vi "util-ui-view.vi"(10 "Page2":enum32{"Map", "Editor", "Calibration"}(ring), 11 "Page1":enum32{"MAIN", "I/O", "ADMIN"}(ring)) -> (2 "Pge2 out":string, 3 "Page1 out":string, 5 "Page1:Page2":string)   [LabVIEW 2024]
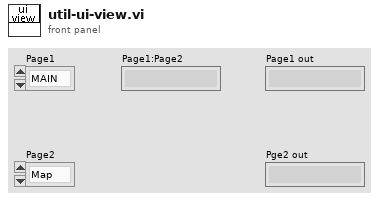
[diagram p1: front panel]
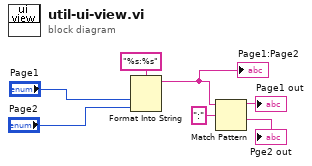
[diagram p0: block diagram]
diagram:
  n1 = Format Into String(format string="%s:%s", "Page1", "Page2") -> (resulting string=w4:string)  [unwired: 2 in, 1 out]
  "Page1:Page2" <- w4
  n2 = Match Pattern(string=w4, regular expression=":") -> (before substring=→"Page1 out":string, after substring=→"Pge2 out":string)  [unwired: 1 in, 2 out]
